vi "start-acquisition.vi"(3 "error in (no error)":errorcluster, 4 "Manufacturer":enum16{"Andor", "Xenics", "unknown"}(ring), 5 "xeva-camref-in":T1) -> (0 "error out":errorcluster, 1 "acqusition started":bool, 2 "xeva-camref-out":T1)   [LabVIEW 2017]
uses:
  <vilib>/Xenics Infrared Solutions/Xeneth LabVIEW API/VIs/Controls/Camara.ctl
  <vilib>/Xenics Infrared Solutions/Xeneth LabVIEW API/Xeneth.lvlib
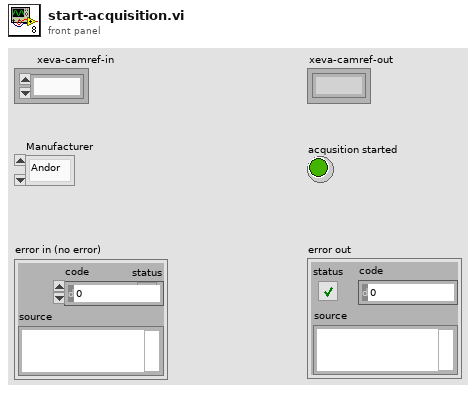
[diagram p1: front panel]
types:
  T1 = typedef "Xeneth.lvlib/Camara.ctl" = refnum<k1>
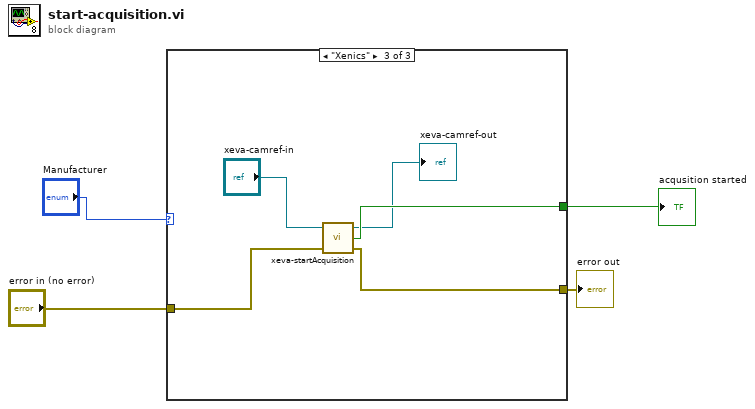
[diagram p0: block diagram]
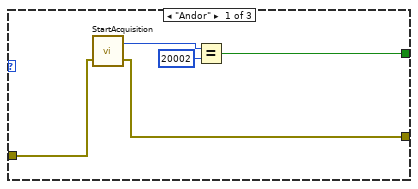
[diagram p2: hidden frame]
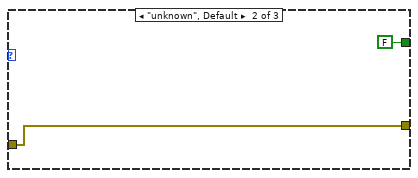
[diagram p3: hidden frame]
diagram:
  n1 = case shown="\"Xenics\"" "Manufacturer" {
    tunnel: [w7 FALSE w16] -> w3
    tunnel: [w6 w10 w15] -> w2
    tunnel: "error in (no error)" -> [w5 w10 w14]
    frame "Andor" {
      n2 = call <userlib>:"StartAcquisition.vi"("error in (no error)"=w5) -> ("error out"=w6:errorcluster, "DLL error code"=w8:u32)  [unwired: 1 in]
      n3 = Equal?(x=w8, y=u32 20002 ("= temperature\naccepted")) -> (x = y?=w7:bool)
    }
    frame "unknown", Default {
    }
    frame "Xenics" {
      n4 = call "xeva-startAcquisition.vi"("error in (no error)"=w14, "xeva-camref"="xeva-camref-in") -> ("error out"=w15:errorcluster, "xeva-acquiring"=w16:bool, "xeva-camref"=→"xeva-camref-out":T1)  [unwired: 1 in]
    }
  }
  "acqusition started" <- w3
  "error out" <- w2
